vi "Assemble QuadViewManager.vi"(8 "Bottom-Right View":refnum<class "IViewable.lvclass">, 9 "Bottom-Left View":refnum<class "IViewable.lvclass">, 10 "Top-Right View":refnum<class "IViewable.lvclass">, 11 "Top-Left View":refnum<class "IViewable.lvclass">) -> (3 "QuadViewManager out":refnum<class "QuadViewManager.lvclass">)   [LabVIEW 2017, in "QuadViewManager.lvlib" / "QuadViewManager.lvclass"]
doc: "<License>\nCopyright © 2017 Composed Systems, LLC | All rights reserved\nwww.composed.io\n\nAuthor: Ethan Stern <ethan.stern@composed.io>\n\nThis software is provided \"AS IS\" WITHOUT WARRANTIES, either express or implied, AND IS FOR EDUCATIONAL PURPOSES ONLY.\n</License>"
uses:
  QuadViewManager.lvclass
  gpm_packages/@cs/mva-viewable/Source/IViewManager/IViewManager/IViewManager.lvclass
  C:/Git/mva-framework/gpm_packages/@cs/mva-viewable/Source/IViewManager/IViewManager/IViewManager.lvclass
  C:/Git/mva-framework/gpm_packages/@cs/mva-viewable/Source/IViewable/IViewable/IViewable.lvclass
  C:/Git/mva-framework/gpm_packages/@cs/mva-viewable/Source/ActorEvents/IEventAggregator/IEventAggregator.lvclass
  C:/Git/mva-framework/gpm_packages/@cs/mva-core/Source/IObserver/IObserver/IObserver.lvclass
  C:/Program Files (x86)/National Instruments/LabVIEW 2017/vi.lib/ActorFramework/Actor/Actor.lvclass
  gpm_packages/@cs/mva-viewable/Source/IViewable/IViewable/IViewable.lvclass
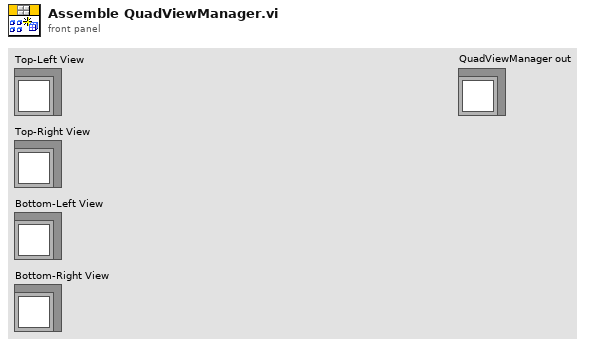
[diagram p1: front panel]
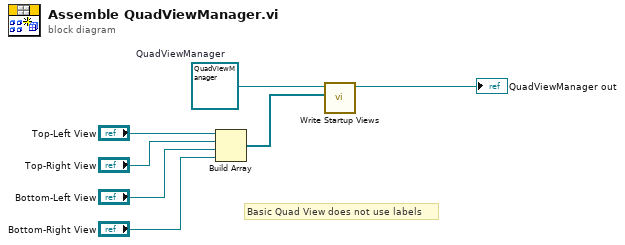
[diagram p0: block diagram]
diagram:
  w7 = refnum<class "QuadViewManager.lvclass"> refnum  # QuadViewManager
  # "Basic Quad View does not use labels"
  n1 = Build Array("Top-Left View", "Top-Right View", "Bottom-Left View", "Bottom-Right View") -> (w1:refnum<class "IViewable.lvclass">[])
  n2 = call "Write Startup Views.vi"("Startup Views"=w1, "IViewManager in"=w7) -> ("IViewManager out"=→"QuadViewManager out":refnum<class "QuadViewManager.lvclass">)  [unwired: 9 in]
